vi "New Driver Input.vi"(8 "error in (no error)":errorcluster, 11 "Driver-Virtual in":refnum<class "Driver-Virtual.lvclass">) -> (0 "error out":errorcluster, 3 "Driver-Virtual out":refnum<class "Driver-Virtual.lvclass">)   [LabVIEW 2013, in "Virtual Systems.lvlib" / "Driver.lvlib" / "Driver-Virtual.lvclass"]
uses:
  Driver-Virtual.lvclass
  Driver-Virtual.lvclass/Driver-Virtual.ctl
  Robot/Logical Systems/Driver/Driver-Logical/Driver.lvclass
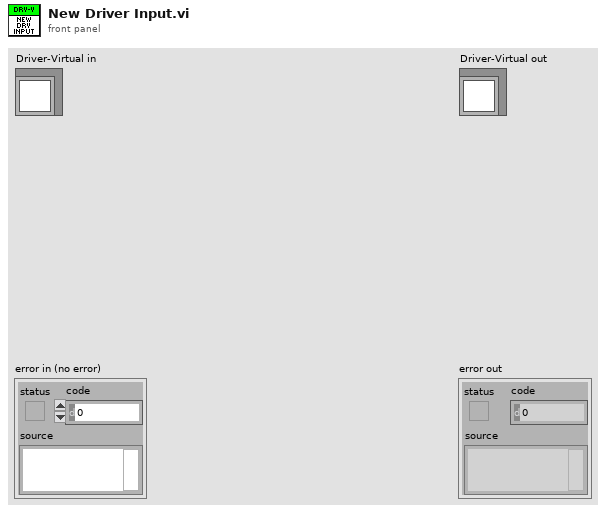
[diagram p1: front panel]
types:
  T1 = typedef "Logical Systems.lvlib/Driver.lvlib/Driver.lvclass/Driver Status.ctl" = cluster{"Current Xbox Controller":T2}
  T2 = typedef "Logical Systems.lvlib/Xbox Controller.lvlib/Xbox Controller.ctl" = cluster{"Left Joystick":T3, "Right Joystick":T3}
  T3 = typedef "Logical Systems.lvlib/Xbox Controller.lvlib/Joystick.ctl" = cluster{"Forward":dbl, "Right":dbl}
  T4 = typedef "Logical Systems.lvlib/Xbox Controller.lvlib/XBox Controller-Logical.lvclass/Joystick.ctl" = cluster{"Forward":dbl, "Right":dbl}
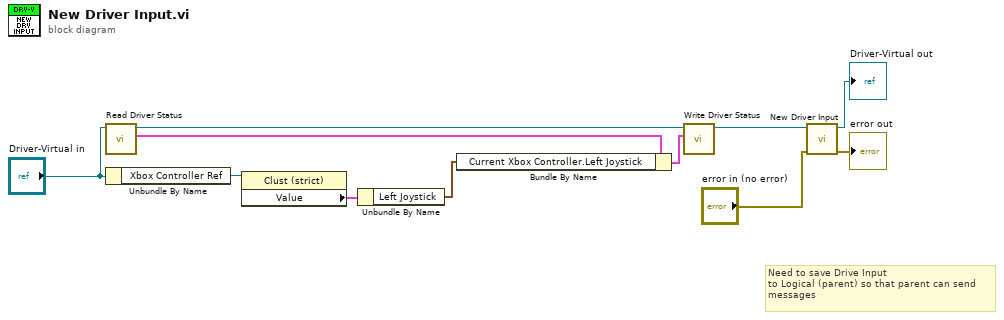
[diagram p0: block diagram]
diagram:
  # "Need to save Drive Input\nto Logical (parent) so that parent can send \nmessages"
  n1 = call-dynamic "Read Driver Status.vi"("Driver in"="Driver-Virtual in") -> ("Driver Status"=w2:T1, "Driver out"=w5:refnum<class "Driver-Virtual.lvclass">)  [unwired: 8 in, 1 out]
  n2 = Unbundle By Name("Driver-Virtual in") -> ("Xbox Controller Ref"=w8:refnum<vi>)
  n3 = property class="Clust (strict)"(reference=w8) -> ("Value"=w7:T2)  [unwired: 1 in, 2 out]
  n4 = Unbundle By Name(w7) -> ("Left Joystick"=w1:T4)
  n5 = Bundle By Name(cluster=w2, "Current Xbox Controller.Left Joystick"=w1) -> (w3:T1)
  n6 = call-dynamic "Write Driver Status.vi"("Driver Status"=w3, "Driver in"=w5) -> ("Driver out"=w4:refnum<class "Driver-Virtual.lvclass">)  [unwired: 8 in, 1 out]
  n7 = call-parent "New Driver Input.vi"("error in (no error)"="error in (no error)", "Driver-Logical in"=w4) -> ("error out"=→"error out":errorcluster, "Driver-Logical out"=→"Driver-Virtual out":refnum<class "Driver-Virtual.lvclass">)  [unwired: 8 in]
